vi "New BetterTreeHandle.vi"(8 "error in (no error)":errorcluster, 10 "TreeBar Picture Ref":refnum<vi>, 11 "TreeRef":refnum<vi>) -> (0 "error out":errorcluster, 3 "BetterTreeHandle out":refnum<class "BetterTreeHandle.lvclass">)   [LabVIEW 2020, in "BetterDragAndDrop.lvlib" / "BetterTreeHandle.lvclass"]
uses:
  BetterTreeHandle.lvclass
  C:/DSCE code/Open-source/betterdraganddrop_GIT/Source/Classes/BetterHandle/BetterHandle.lvclass
  BetterTreeHandle.lvclass/BetterTreeHandle.ctl
  BetterHandle/BetterHandle.lvclass/BetterHandle.ctl
  BetterHandle/Write TreeBar.vi
  BetterTreeBar/BetterHorizontalBar.lvclass
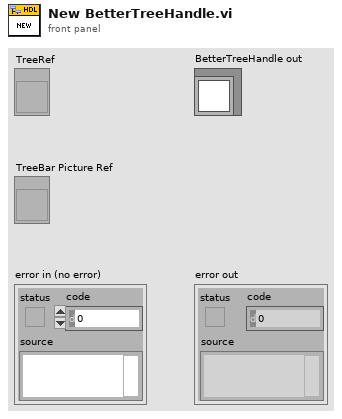
[diagram p1: front panel]
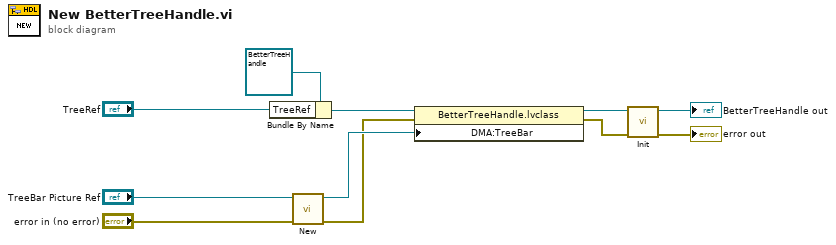
[diagram p0: block diagram]
diagram:
  n1 = Bundle By Name(cluster=refnum<class "BetterTreeHandle.lvclass"> refnum ("BetterTreeHandle out"), "TreeRef"="TreeRef") -> (w7:refnum<class "BetterTreeHandle.lvclass">)
  n2 = call "New.vi"("error in (no error)"="error in (no error)", "Picture Ref"="TreeBar Picture Ref") -> ("error out"=w4:errorcluster, "BetterTreeBar out"=w6:refnum<class "BetterHorizontalBar.lvclass">)  [unwired: 8 in]
  n3 = property class="BetterTreeHandle.lvclass"(reference=w7, error in=w4, "DMA:TreeBar"=w6) -> (reference out=w5:refnum<class "BetterTreeHandle.lvclass">, error out=w3:errorcluster)
  n4 = call-dynamic "Init.vi"("error in (no error)"=w3, "BetterTreeHandle in"=w5) -> ("error out"=→"error out":errorcluster, "BetterTreeHandle out"=→"BetterTreeHandle out":refnum<class "BetterTreeHandle.lvclass">)  [unwired: 8 in]
